vi "BeadCoolerFixedZ(SubVI).vi"(0 "hp coeff band":i32[](array[numeric])=[-850883994, 1909449570, 958518847, -975456236, 2033039520, 1020559395], 1 "lp coeff band":i32[](array[numeric])=[-955995012, 2025731616, 1001305, -1023351008, 2092954700, 1034533], 2 "ig":fxp<+/-,24,-4>, 3 "dg":fxp<+/-,24,12>, 4 "load (F)":bool, 5 "pg":fxp<+/-,24,12>, 6 "dg band":fxp<+/-,24,12>, 7 "Notch coeff 1":i32[](array[numeric])=[-1060332860, 1067037342, -2129863576], 9 "Notch coeff 2":i32[](array[numeric])=[-1060332860, 1067037342, -2129863576], 10 "AI0":i16, 12 "Dc Pos":i16, 13 "Upper lim":fxp<+/-,16,16>, 16 "lp coeff":i32[](array[numeric])=[1008310688, 32715568], 17 "Lower lim":fxp<+/-,16,16>, 18 "final filter coeff":i32[](array[numeric])=[-955995012, 2025731616, 1001305, -1023351008, 2092954700, 1034533], 23 "hp coeff":i32[](array[numeric])=[946630756, 1010186290]) -> (25 "Output":fxp<+/-,16,16>, 26 "accurm reset":bool, 27 "accum out":fxp<+/-,37,37>)   [LabVIEW 2018]
uses:
  <vilib>/rvi/FXPMathLib/basic elements/FxpIntAccumulator/subVIs/nifxpmath_IntAccumulator_SimConfig.ctl
  <vilib>/rvi/FXPMathLib/basic elements/FxpIntAccumulator/simVIs/DllFxpIntAccumulator_sub.vi
  <vilib>/rvi/FXPMathLib/FxpInterpret/XNode/nifxpmath_Interpret.xnode
  <vilib>/rvi/FXPMathLib/basic elements/FxpIntAccumulator/XNode/nifxpmath_IntAccumulator.xnode
  <vilib>/rvi/Analysis/measure/butterworth/XNode/niFpgaButterworthFilter.xnode
  <vilib>/rvi/Analysis/measure/notch/XNode/niFpgaNotchFilter.xnode
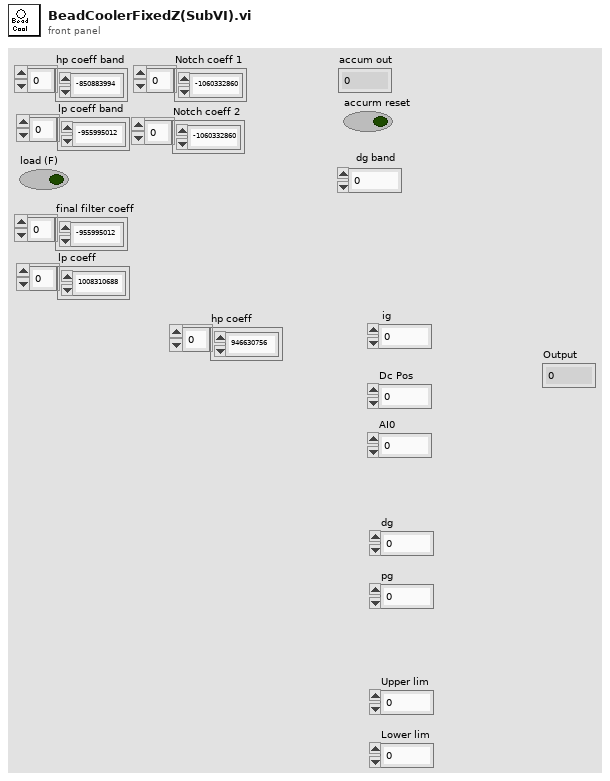
[diagram p1: front panel]
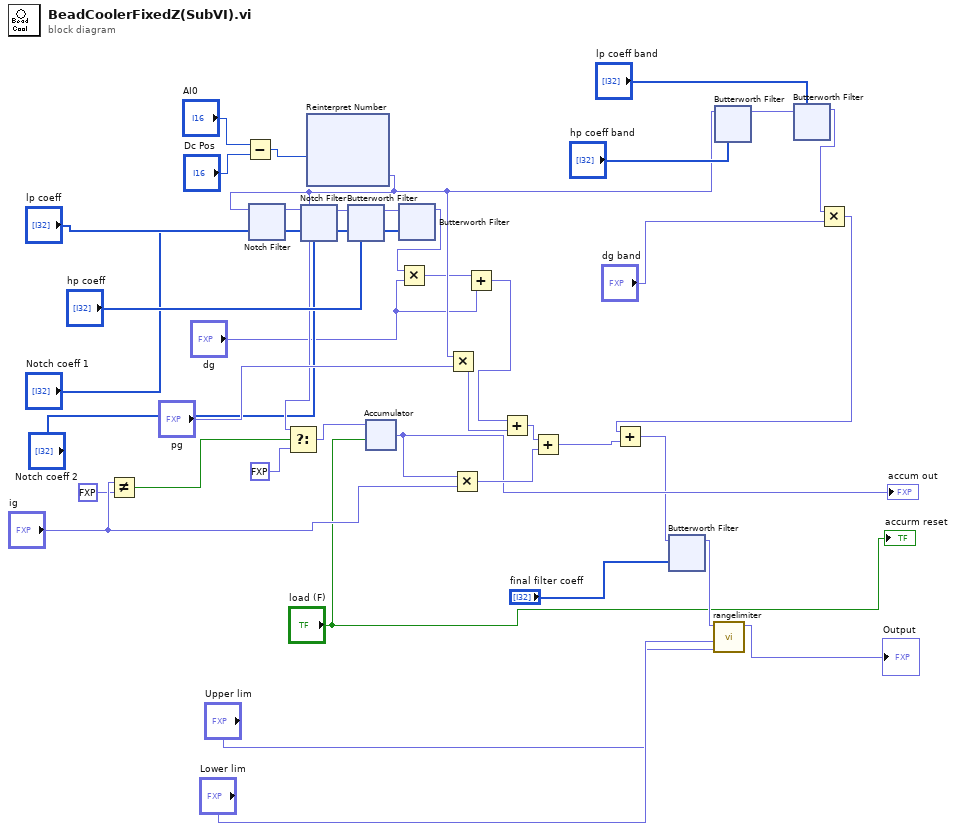
[diagram p0: block diagram]
diagram:
  n1 = Not Equal?(x="ig", y=fxp<+/-,24,6> 0.0) -> (x != y?=w23:bool)
  n2 = Subtract(x="AI0", y="Dc Pos") -> (x-y=w34:i16)
  n3 = xnode "Reinterpret Number"("x"=w34) -> ("y"=w7:fxp<+/-,16,16>)
  n4 = xnode "Notch Filter"("input data"=w7, "scaled coefficients"="Notch coeff 1") -> ("output data"=w6:fxp<+/-,16,16>)  [unwired: 1 in]
  n5 = Select(t=w7, s=w23, f=fxp<+/-,16,16> 0.0) -> (s? t:f=w25:fxp<+/-,16,16>)
  n6 = xnode "Notch Filter"("input data"=w6, "scaled coefficients"="Notch coeff 2") -> ("output data"=w5:fxp<+/-,16,16>)  [unwired: 1 in]
  n7 = xnode "Butterworth Filter"("input data"=w5, "scaled coefficients"="hp coeff") -> ("output data"=w27:fxp<+/-,16,16>)  [unwired: 1 in]
  n8 = xnode "Accumulator"("x"=w25, "load (F)"="load (F)") -> ("s"=w29:fxp<+/-,37,37>)  [unwired: 3 in, 1 out]
  "accum out" <- w29
  n9 = xnode "Butterworth Filter"("input data"=w27, "scaled coefficients"="lp coeff") -> ("output data"=w26:fxp<+/-,16,16>)  [unwired: 1 in]
  n10 = Multiply(x=w26, y="dg") -> (x*y=w2:fxp<+/-,18,16>)
  n11 = Multiply(x=w7, y="pg") -> (x*y=w39:fxp<+/-,18,16>)
  n12 = Multiply(x=w29, y="ig") -> (x*y=w30:fxp<+/-,18,16>)
  n13 = Add(x=w2, y="dg") -> (x+y=w1:fxp<+/-,29,17>)
  n14 = Add(x=w1, y=w39) -> (x+y=w31:fxp<+/-,18,16>)
  n15 = Add(x=w31, y=w30) -> (x+y=w16:fxp<+/-,16,16>)
  n16 = xnode "Butterworth Filter"("input data"=w7, "scaled coefficients"="hp coeff band") -> ("output data"=w20:fxp<+/-,16,16>)  [unwired: 1 in]
  n17 = xnode "Butterworth Filter"("input data"=w20, "scaled coefficients"="lp coeff band") -> ("output data"=w19:fxp<+/-,16,16>)  [unwired: 1 in]
  n18 = Multiply(x=w19, y="dg band") -> (x*y=w17:fxp<+/-,18,16>)
  n19 = Add(x=w17, y=w16) -> (x+y=w13:fxp<+/-,16,16>)
  n20 = xnode "Butterworth Filter"("input data"=w13, "scaled coefficients"="final filter coeff") -> ("output data"=w12:fxp<+/-,16,16>)  [unwired: 1 in]
  n21 = call "rangelimiter.vi"("Upper lim"="Upper lim", "Lower lim"="Lower lim", "Input"=w12) -> ("Output"=→"Output":fxp<+/-,16,16>)  [unwired: 8 in]
  "accurm reset" <- "load (F)"
